vi "Robot_Targeting_adjustment.vi"   [LabVIEW 2017]
uses:
  <vilib>/addons/control/pid/NI_PID_pid.lvlib
  <vilib>/addons/control/pid/pid.llb/PID (DBL).vi
panel:
  # ".7\n-.7"
  # "1\n-1"
  # ".5\n-.5"
  # "Rotation"
  # "Strafe"
  # "Forward back"
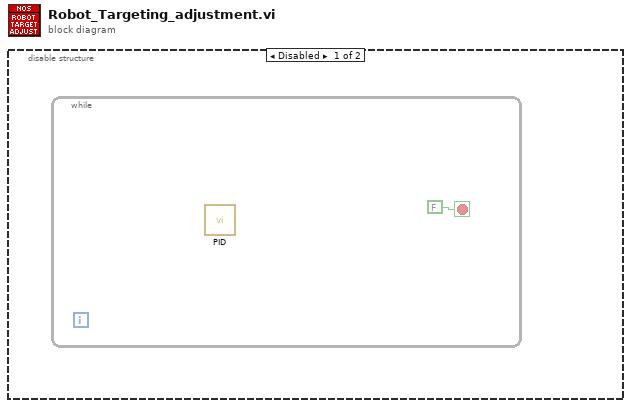
[diagram p0: block diagram]
diagram:
  n1 = disable-structure shown="Disabled" {
    frame Disabled {
      n2 = while {
        stop <- FALSE stop-if-true
        n3 = call-poly <vilib>:"PID.vi"() -> ()  [unwired: 10 in, 2 out]
      }
    }
    frame Enabled {
    }
  }
